vi "CAN Filter Messages.vi"(7 "Mode":u8, 8 "error in (no error)":errorcluster, 9 "ToID":u32, 10 "FromID":u32, 11 "Channel":u16) -> (0 "error out":errorcluster, 3 "function return":u32)   [LabVIEW 2017, in "PCANBasic_eX.lvlib"]
doc: "TPCANStatus __stdcall CAN_FilterMessages(\n TPCANHandle Channel, \n DWORD FromID, \n DWORD ToID, \n TPCANMode Mode);"
uses:
  PCANBasic_eX.lvlib
  PCANBasic.dll
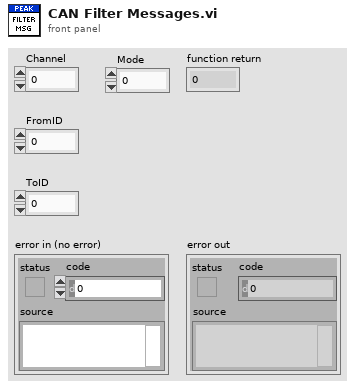
[diagram p1: front panel]
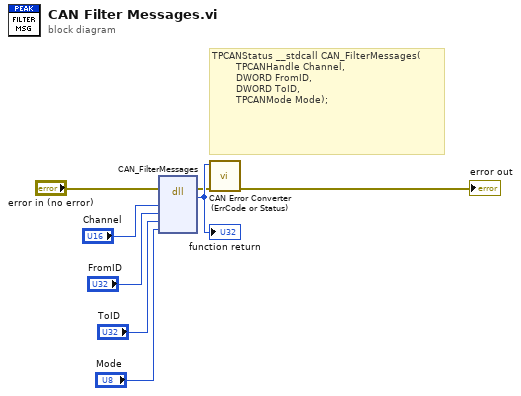
[diagram p0: block diagram]
diagram:
  # "TPCANStatus __stdcall CAN_FilterMessages(\n        TPCANHandle Channel, \n        DWORD FromID, \n        DWORD ToID, \n        TPCANMode Mode);"
  n1 = dll-call lib="PCANBasic.*" fn="CAN_FilterMessages"(error in="error in (no error)", "Channel"="Channel", "FromID"="FromID", "ToID"="ToID", "Mode"="Mode") -> (error out=w2:errorcluster, w8:u32)  [unwired: 6 in, 1 out]
  "function return" <- w8
  n2 = call "CAN Error Converter (ErrCode or Status).vi"("error in (no error)"=w2, "error code"=w8) -> ("error out"=→"error out":errorcluster)  [unwired: 9 in]
